vi "Joystick_Normalize.vi"(7 "Power":sgl=100.0, 11 "Joystick In":i8) -> (3 "Norm Out":sgl)   [LabVIEW 2012]
doc: "converts joystick input to motor power."
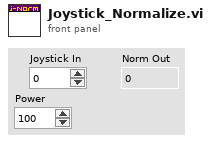
[diagram p1: front panel]
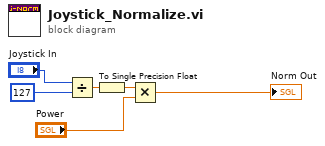
[diagram p0: block diagram]
diagram:
  n1 = Divide(x="Joystick In", y=i8 127) -> (x/y=w3:dbl)
  n2 = To Single Precision Float(number=w3) -> (single precision float=w1:sgl)
  n3 = Multiply(x=w1, y="Power") -> (x*y=→"Norm Out":sgl)
